vi "Day 20-Process Image.vi"(9 "Previous \"Infinity\" value":bool, 10 "Lookup Array":bool[](array[boolean]), 11 "Image in":bool[][](array[boolean])) -> (1 "New \"Infinity\" Value":bool, 3 "Image out":bool[][](array[boolean]))   [LabVIEW 2021]
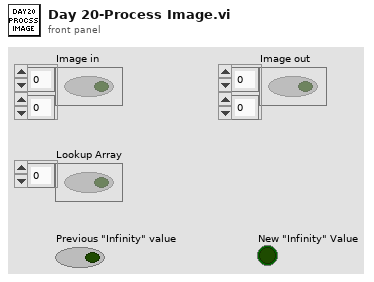
[diagram p1: front panel]
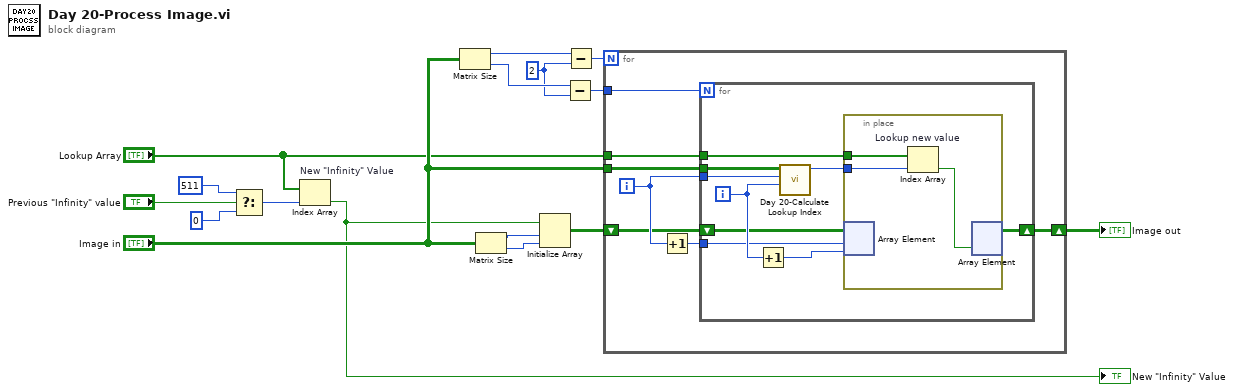
[diagram p0: block diagram]
diagram:
  w13 = 2
  n1 = Select(t=511, s="Previous \"Infinity\" value", f=0) -> (s? t:f=w4:i32)
  n2 = Index Array "New \"Infinity\" Value"(array="Lookup Array", index=w4) -> (element=w2:bool)
  "New \"Infinity\" Value" <- w2
  n3 = Matrix Size(0:"Image in") -> (1:w14:i32, 2:w15:i32)
  n4 = Matrix Size(0:"Image in") -> (1:w8:i32, 2:w9:i32)
  n5 = Initialize Array(w2, w8, w9) -> (w10:bool[][])
  n6 = Subtract(x=w15, y=w13) -> (x-y=w12:i32)
  n7 = Subtract(x=w14, y=w13) -> (x-y=w11:i32)
  n8 = for {
    N: w11 -> [_]
    tunnel: "Image in" -> [w22]
    tunnel: w12 -> [w21]
    tunnel: "Lookup Array" -> [w20]
    shift-right: [w17] -> w7
    shift-left: w10 -> [w18]
    i -> [w23]
    n9 = Increment(x=w23) -> (x+1=w19:i32)
    n10 = for {
      N: w21 -> [_]
      tunnel: w22 -> [w31]
      tunnel: w19 -> [w25]
      tunnel: w20 -> [w30]
      shift-right: [w27] -> w17
      shift-left: w18 -> [w28]
      tunnel: w23 -> [w26]
      i -> [w32]
      n11 = Increment(x=w32) -> (x+1=w24:i32)
      n12 = call "Day 20-Calculate Lookup Index.vi"("Left of Subgrid"=w32, "Top of Subgrid"=w26, "Array in"=w31) -> ("Lookup Index"=w29:u32)  [unwired: 8 in]
      n13 = in-place {
        in-place-border: w30 -> [w35]
        in-place-border: w29 -> [w34]
        n14 = in-place-array #1(w28, w25, w24) -> ()  [unwired: 1 out]
        n15 = Index Array "Lookup new value"(array=w35, index=w34) -> (element=w33:bool)
        n16 = in-place-array #1(w33) -> (w27:bool[][])  [unwired: 2 out]
      }
    }
  }
  "Image out" <- w7
